vi "SDCP - Standard Message Frame - Parameter Encode Test.vi"() -> ()   [LabVIEW 2020]
uses:
  Typedefs/SDCP - SMF parameter descriptors.ctl
  Typedefs/SDCP - Standard Message Frames FGV - Commands.ctl
panel:
  out "Encoded message frame 2":u8[](array[numeric]) format="%x"
  in  "SMF descriptor in 2":T1
  in  "Value in 2":string
  out "Encoded message frame 1":u8[](array[numeric]) format="%x"
  in  "Value in 1":string
  in  "SMF descriptor in 1":T1
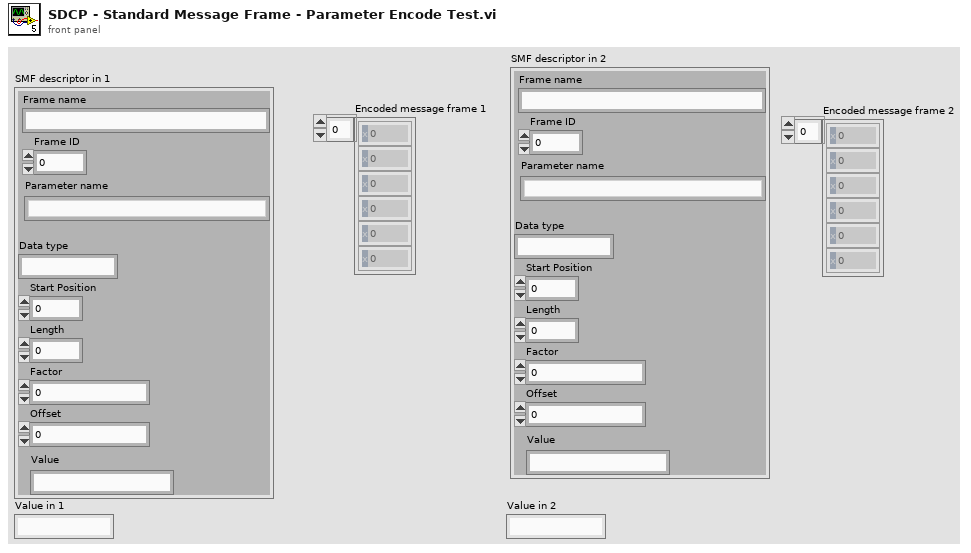
[diagram p1: front panel]
types:
  T1 = typedef "SDCP - SMF parameter descriptors.ctl" = cluster{"Frame name":string, "Frame ID":i32, "Data type":string, "Start Position":i32, "Length":i32, "Factor":dbl, "Offset":dbl, "Parameter name":string, "Value":string}
  T2 = typedef "SDCP - Standard Message Frames FGV - Commands.ctl" = enum16{"Reset", "Read", "Write", "Set Priority"}
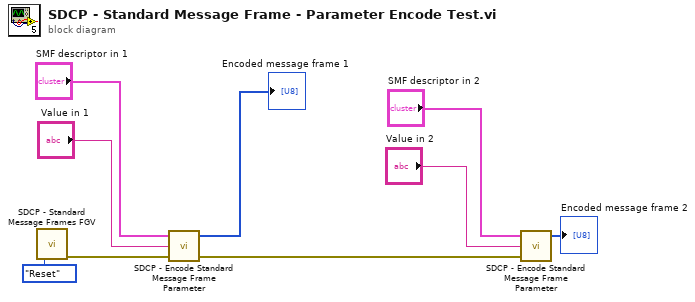
[diagram p0: block diagram]
diagram:
  n1 = call "SDCP - Standard Message Frames FGV.vi"("Command"=SDCP_-_Standard_Message_Frames_FGV_-_Commands."Reset") -> ("error out"=w9:errorcluster)  [unwired: 5 in, 2 out]
  n2 = call "SDCP - Encode Standard Message Frame Parameter.vi"("error in (no error)"=w9, "Value in"="Value in 1", "SMF descriptor in"="SMF descriptor in 1") -> ("error out"=w5:errorcluster, "Encoded message frame"=→"Encoded message frame 1":u8[])  [unwired: 1 in]
  n3 = call "SDCP - Encode Standard Message Frame Parameter.vi"("error in (no error)"=w5, "Value in"="Value in 2", "SMF descriptor in"="SMF descriptor in 2") -> ("Encoded message frame"=→"Encoded message frame 2":u8[])  [unwired: 1 in, 1 out]
